vi "Main v1.7.vi"() -> ()   [LabVIEW 2017]
doc: "v0.85:\n- Counts for rejects and total\n\nv0.5:\n\n- Added Reject to Manual Mode\n- Send reject pallet cluster during manual mode\n- Run continuous manual happens only when no error has occured"
uses:
  Controls/Main Tabs v0.1.ctl
  Controls/Auto.ctl
  RT/Controls/Auto Delays.ctl
  RT/Controls/Auto Times.ctl
  support/Controls/General Para.ctl
  support/Message Queue/Message Cluster.ctl
  Controls/UI Data.ctl
  support/Controls/Auto Stats.ctl
  Controls/Logging FGV.ctl
  support/Message Queue/Enqueue Message (Single).vi
  GV/Maintenance GV.vi
  <vilib>/Utility/error.llb/Error Cluster From Error Code.vi
  <vilib>/ErrorRing/Error Ring.xnode
  support/Message Queue/Message Queue.lvlib
  support/User Event - Stop/User Event - Stop.lvlib
panel:
  in  "dup Message Queue":refnum<queue>
  out "path":path
  in  "General Para 2":T1={"Max. Cons."=5.0, "Offset 1"=0.0, "Offset 2"=0.0, "Offset 3"=0.0, "Offset 4"=-0.6, "OutputPause"=500.0, "RejectPause"=500.0} caption="General Para" {"Offset 4" format="%.2f"; "Offset 3" format="%.2f"; "Offset 2" format="%.2f"; "Offset 1" format="%.2f"}
  in  "Auto Para 2":T2={"Agitator Delays"=[250, 600], "TF Delays"=[400, 800, 2, 8000], "Insertion Delays"=[100, 400], "Cutting Delays"=[200, 300, 50], "PF Delays"=[300, 8000], "Measur. Delays"=[200.0, 188.9, 1.0], "Reject Delays"=[500], "BF Delays"=[1000, 1000]}
  out "Shutdown?":bool
  out "Boolean 8":bool
  out "Boolean 7":bool
  out "Boolean 6":bool
  out "Boolean 5":bool
  out "Boolean 4":bool
  out "Boolean 3":bool
  out "Boolean 2":bool
  out "Boolean":bool
  in  "Reject Pallets":T3
  out "Date-Time":string caption="Dip-Tube Assembly Automation (HMI) v1.6"
  out "Main Tab":T4
  in  "All IOs":bool
  in  "Autocycle":T5
  in  "Manual":bool
  in  "Parameters":bool
  in  "Maintenance":bool
  in  "Info":bool
  in  "General Para":T1={"Max. Cons."=5.0, "Offset 1"=0.0, "Offset 2"=0.0, "Offset 3"=0.0, "Offset 4"=0.0, "OutputPause"=0.0, "RejectPause"=0.0} {"Offset 4" format="%.2f"; "Offset 3" format="%.2f"; "Offset 2" format="%.2f"; "Offset 1" format="%.2f"}
  in  "BF Para":cluster{"Delay 1":u32, "Delay 2":u32}={"Delay 1"=1000, "Delay 2"=1000}
  in  "Reject Para":cluster{"Delay":u32}={"Delay"=400}
  in  "Meas. Para":T6={"Delay"=500.0, "Mean Length"=188.9, "Tolerance"=1.0}
  in  "PF Para":cluster{"Delay":u32, "Timeout":u32}={"Delay"=1000, "Timeout"=1000}
  in  "Tube Feeder Para":T7={"Delay"=400, "Delay 2"=250, "Max Attempts"=250, "Timeout"=8000}
  in  "Cutting Para":T8={"Delay"=400, "Delay 2"=250, "Delay 3"=250}
  in  "Agitator Para":cluster{"Delay":u32, "Timeout":u32}={"Delay"=400, "Timeout"=250}
  in  "Insertion Para":cluster{"Delay 1":u32, "Delay 2":u32}={"Delay 1"=1000, "Delay 2"=1000}
  in  "Save Para":bool
  in  "Home Para":bool
  out "OEE":dbl format="%#.1f"
  out "QUA":dbl=100.0 min=0.0 max=100.0 step=0.1
  in  "Ideal Time":dbl=2.0 min=0.0 max=100.0 step=0.1
  in  "AVL":dbl=100.0 min=0.0 max=100.0 step=0.1
  out "Rejects 2":u32 caption="Rejects"
  in  "Reset MCount":bool
  in  "Enable BF?":bool
  in  "Enable Agitate?":bool
  in  "Enable Reject?":bool
  in  "Toggle Motor":bool
  in  "Continuous?":bool
  in  "Enable Measure?":bool
  in  "Enable Index?":bool
  in  "Enable PF?":bool
  in  "Manual Para":T2={"Agitator Delays"=[400, 250], "TF Delays"=[700, 800, 2], "Insertion Delays"=[100, 500], "Cutting Delays"=[300, 300, 100], "PF Delays"=[250, 30000], "Measur. Delays"=[500.0, 188.9, 1.0], "Reject Delays"=[500], "BF Delays"=[1000, 1000]}
  in  "Enable Cutting?":bool
  in  "Enable Insertion?":bool
  in  "Run Manual":bool
  in  "Enable TF?":bool
  in  "Home Manual":bool
  out "Status 2":T10
  out "Measurements":T11 {"Height 1" format="%#.2f"; "Height 2" format="%#.2f"; "Height 3" format="%#.2f"; "Height 4" format="%#.2f"}
  out "Output Count":u32 caption="Output\nCount"
  out "PRF":dbl=100.0 min=0.0 max=100.0 step=0.1
  in  "ResetRejectCount":bool
  in  "ResetGoodCount":bool
  out "RejectPause":u32 caption="Reject Parts"
  out "GoodPause":u32 caption="Good Parts"
  in  "End Cycle":bool
  out "Statuses":string[][](table)
  in  "All IO":bool
  in  "Stats":bool
  in  "Home AC":bool
  out "Status":string
  out "Good":u32 format="%06.0f"
  out "Cycle Time":dbl format="%0.2f"
  out "Rejects":u32 format="%05.0f"
  in  "View Log":bool
  out "Total Count 2":u32 caption="Total Count"
  out "Avg. Time":dbl caption="Avg. Cycle Time (s)" format="%#.3f"
  out "Output Chart":cluster{"Good Parts":u32, "Reject Parts":u32}(graph)
  out "Reject Count":u32
  out "Good Count":u32
  out "Total Time":dbl caption="Effective Cycle Time (s)" format="%#.3f"
  out "Time Chart":T12(graph)
  out "OEE Chart":T13(graph)
  out "Timestamp":string caption="Date & Timestamp"
  out "Latest Measure.":T14 caption="Latest Measurements" {"Length 1 (mm)" format="%#.2f"}
  out "Auto Times":T9
  in  "Back Stats":bool
  out "OEE 2":T13 caption="Latest Measurements" {"AVL" format="%#.1f"; "PRF" format="%#.1f"; "QUA" format="%#.1f"; "OEE" format="%#.1f"}
  out "Measurement Chart":T15(graph)
  in  "Home IOs":bool
  in  "Back IO":bool
  out "IAS 4":dbl format="%#.3f"
  out "IAS 3":dbl format="%#.3f"
  out "IAS 2":dbl format="%#.3f"
  out "IAS 1":dbl format="%#.3f"
  out "DI 1":T16
  out "DI 2":T17
  out "DO 1":T18
  in  "Exit":bool
  in  "Shutdown":bool
  # "HARMONY VISION DIP-TUBE ASSEMBLY AUTOMATION"
  # "Auto-Pause after"
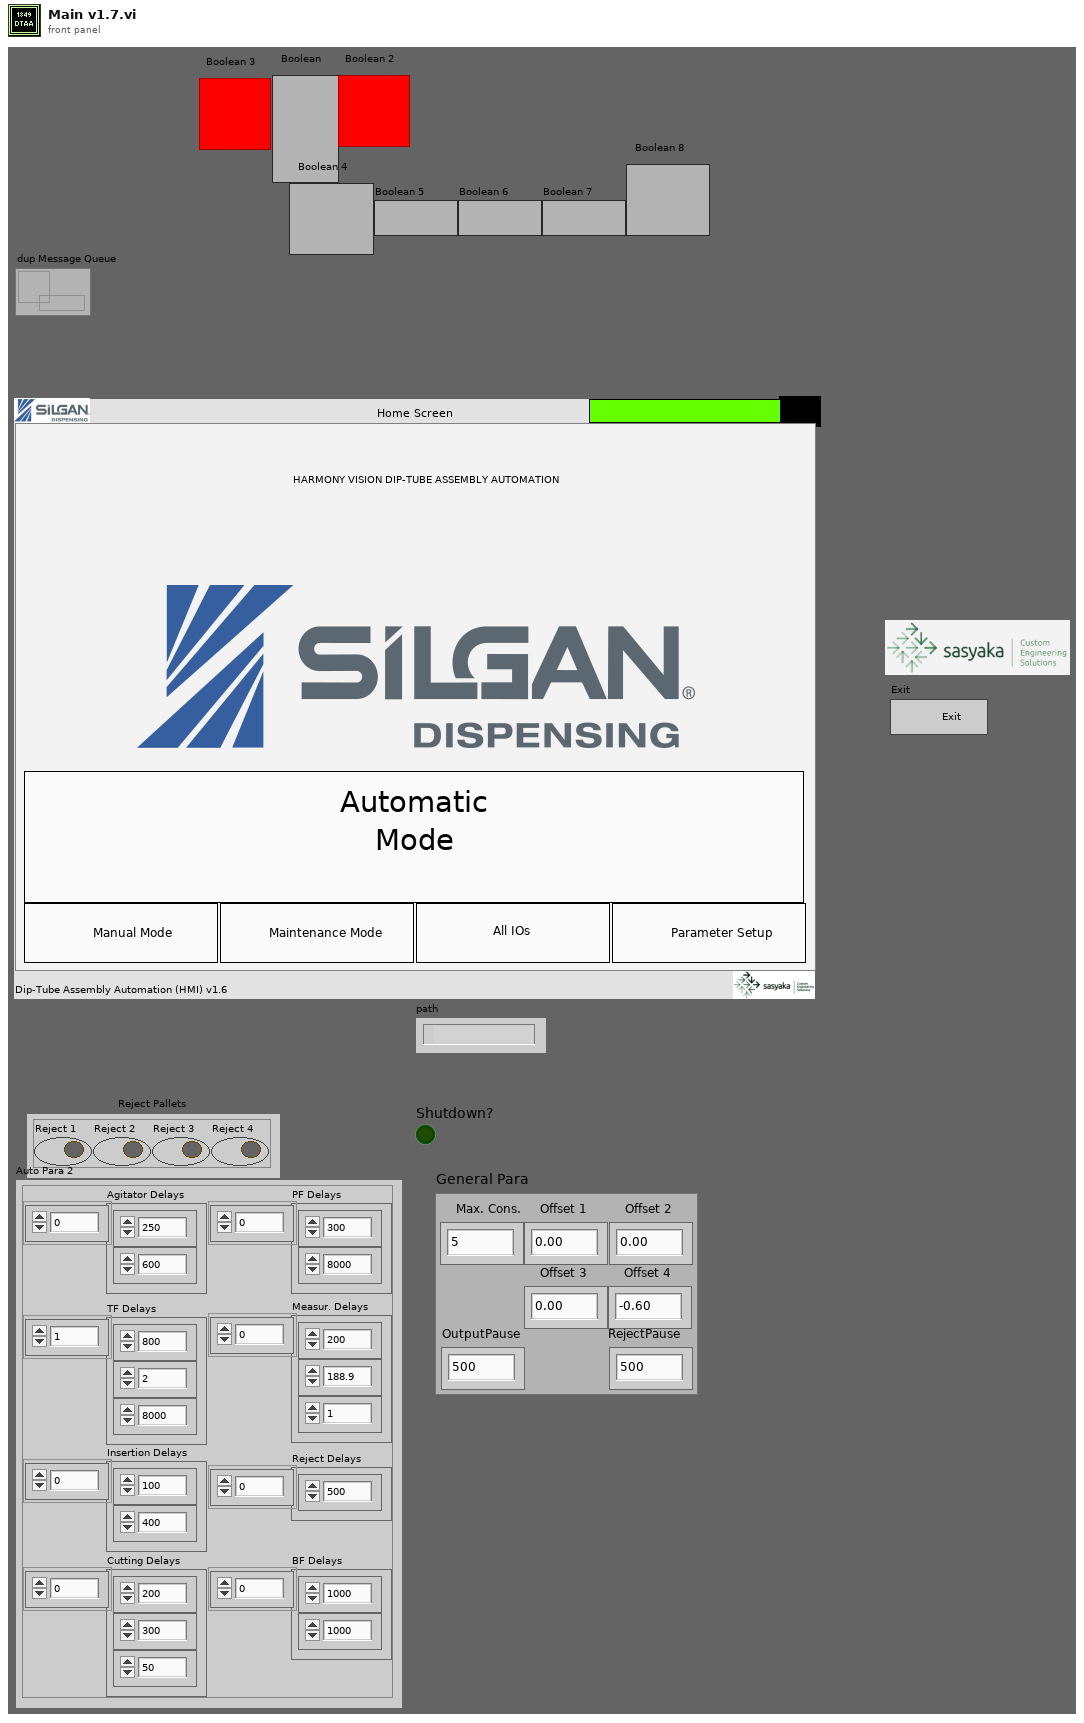
[diagram p1: front panel]
types:
  T1 = typedef "General Para.ctl" = cluster{"Max. Cons.":dbl, "Offset 1":dbl, "Offset 2":dbl, "Offset 3":dbl, "Offset 4":dbl, "OutputPause":dbl, "RejectPause":dbl}
  T2 = typedef "Auto Delays.ctl" = cluster{"Agitator Delays":u32[], "TF Delays":u32[], "Insertion Delays":u32[], "Cutting Delays":u32[], "PF Delays":u32[], "Measur. Delays":dbl[], "Reject Delays":u32[], "BF Delays":u32[]}
  T3 = cluster{"Reject 1":bool, "Reject 2":bool, "Reject 3":bool, "Reject 4":bool}
  T4 = typedef "Main Tabs v0.1.ctl" = enum32{"Home Screen", "Parameter Setup", "Manual Mode", "Autocycle", "Autocycle Statistics", "Autocycle IOs"}
  T5 = typedef "Auto.ctl" = bool
  T6 = cluster{"Delay":dbl, "Mean Length":dbl, "Tolerance":dbl}
  T7 = cluster{"Delay":u32, "Delay 2":u32, "Max Attempts":u32, "Timeout":u32}
  T8 = cluster{"Delay":u32, "Delay 2":u32, "Delay 3":u32}
  T9 = typedef "Auto Times.ctl" = cluster{"Index Time":u32, "TF Time":u32, "Insertion Time":u32, "Cutting Time":u32, "PF Time":u32, "Meas. Time":u32, "Reject Time":u32}
  T10 = cluster{"Auto Times":T9, "error out":errorcluster}
  T11 = cluster{"Height 1":dbl, "Height 2":dbl, "Height 3":dbl, "Height 4":dbl}
  T12 = cluster{"Index":dbl, "TF":dbl, "Insert":dbl, "Cutting":dbl, "PF":dbl, "Measure.":dbl, "Reject":dbl, "Avg. Cycle Time":dbl}
  T13 = cluster{"AVL":dbl, "PRF":dbl, "QUA":dbl, "OEE":dbl}
  T14 = cluster{"Length 1 (mm)":dbl, "Pallet 2 (mm)":dbl, "Pallet 3 (mm)":dbl, "Pallet 4 (mm)":dbl}
  T15 = cluster{"1":dbl, "2":dbl, "3":dbl, "4":dbl, "4":dbl, "4":dbl}
  T16 = cluster{"Machine_ON":bool, "E_stop ":bool, "SW_Pressure":bool, "SW_Start ":bool, "SW_Reset":bool, "SW_Stop":bool, "SW_Door":bool, "RS_Index_Rotary_CW":bool, "RS_Index_Rotary_CCW":bool, "RS_Index_Stopper _Rear":bool, "RS_Index_Output_Separator_Rear":bool, "PES_Index_Pallet_Sensor":bool, "PES_Index_Output_Part Sensor":bool, "ICS_BF_Low_Level_1":bool, "ICS_BF_Low_Level_2":bool, "ICS_BF_Pump_CNVR_Full_1":bool, "ICS_BF_Pump_CNVR_Full_2":bool, "ICS_BF_Pump_CNVR_Full_3":bool, "ICS_BF_Pump_CNVR_Full_4":bool, "PES_PC_Pump Presence_1":bool, "PES_PC_Pump Presence_2":bool, "PES_PC_Pump Presence_3":bool, "PES_PC_Pump Presence_4":bool, "RS_PC_Gating_Front":bool, "PES_Pump_Interference":bool, "PES_TF_Low_Level":bool, "PES_Tube Presence_1":bool, "PES_Tube Presence_2":bool, "PES_Tube Presence_3":bool, "PES_Tube Presence_4":bool, "DI1.30":bool, "DI1.31":bool}
  T17 = cluster{"RS_Agitatator_1_Rear ":bool, "RS_Agitatator_2_Rear ":bool, "RS_TF_Gating CYL_Rear":bool, "RS_Insertion_1_Rear":bool, "RS_Insertion_1_Front":bool, "RS_Insertion _2_Rear":bool, "RS_Insertion _2_Front":bool, "RS_Insertion _3_Rear":bool, "RS_Insertion _3_Front":bool, "RS_Insertion _4_Rear":bool, "RS_Insertion _4_Front":bool, "RS_Insertion_Clamp_Rear":bool, "RS_Cutting_Rear":bool, "RS_Cutting_Clamp _Rear":bool, "RS_Measurement_1_Rear":bool, "RS_Measurement_2_Rear":bool, "RS_Measurement_3_Rear":bool, "RS_Measurement_4_Rear":bool, "DI2.18":bool, "RS_Rejection_1_Rear":bool, "RS_Rejection_2_Rear":bool, "RS_Rejection_3_Rear":bool, "RS_Rejection_4_Rear":bool, "DI2.23":bool, "DI2.24":bool, "DI2.25":bool, "DI2.26":bool, "DI2.27":bool, "DI2.28":bool, "DI2.29":bool, "DI2.30":bool, "DI2.31":bool}
  T18 = cluster{"TL_Red":bool, "TL_Orange":bool, "TL_Green":bool, "TL_Buzzer":bool, "SOL_Index_Rotary_CW":bool, "SOL_Index_Rotary_CCW":bool, "SOL_Index_Stopper_Rear":bool, "SOL_OutputSeparator_Rear":bool, "Bowl  Feeder_ ON 1":bool, "Pump_CNVR_Motor _ON":bool, "SOL_PC_Gating_CYL_Rear":bool, "SOL_Tube_Feed_Agitatator":bool, "SOL_Tube_Feed_Gating_CYL":bool, "SOL_Insertion _CYL":bool, "SOL_Insertion_Clamp_CYL":bool, "SOL_Cutting_CYL":bool, "SOL_Cutting_Clamp_CYL":bool, "SOL_Insertion_Air_Nozzle":bool, "SOL_Measurement_CYL":bool, "DO1.19":bool, "SOL_Rejection CYL_1":bool, "SOL_Rejection CYL_2":bool, "SOL_Rejection CYL_3":bool, "SOL_Rejection CYL_4":bool, "Bowl  Feeder_ ON 2":bool, "SOL_BF_BlowerON":bool, "SOL_BF1_Track1":bool, "SOL_BF1_Track2":bool, "SOL_BF2_Track1":bool, "SOL_BF2_Track2":bool, "DO1.30":bool, "DO1.31":bool}
  T19 = typedef "UI Data.ctl" = cluster{"Main Tab":refnum<vi>}
  T20 = typedef "Message Queue.lvlib/All Message Queues.ctl" = cluster{"UI":refnum<queue>}
  T21 = enum8{"Enabled", "Disabled", "Disabled and Grayed Out"}
  T22 = cluster{"Array":string[][], "Machine Status":string}
  T23 = typedef "Logging FGV.ctl" = enum16{"Start Shift", "Log Index", "Read Shift", "Close Shift"}
  T24 = typedef "Auto Stats.ctl" = cluster{"Time-Stamp":timestamp, "Auto Times":T9, "Measurements":cluster{"1":dbl, "2":dbl, "3":dbl, "4":dbl}, "Outputs":cluster{"Good Parts":u32, "Reject Parts":u32}, "Cycle Time":dbl, "Remarks":string}
  T25 = cluster{"Auto Times":T9, "Results":cluster{"Measurements":cluster{"1":dbl, "2":dbl, "3":dbl, "4":dbl}, "Reject Pallets":cluster{"Reject 1":bool, "Reject 2":bool, "Reject 3":bool, "Reject 4":bool}}, "OutputCount":u32, "error out":errorcluster}
  T26 = enum8{"Information", "Error", "Successful", "Tips"}
  T27 = cluster{"Agitator Delays[0]":u32, "Agitator Delays[1]":u32}
  T28 = cluster{"TF Delays[0]":u32, "TF Delays[1]":u32, "TF Delays[2]":u32, "TF Delays[3]":u32}
  T29 = cluster{"Insertion Delays[0]":u32, "Insertion Delays[1]":u32}
  T30 = cluster{"Cutting Delays[0]":u32, "Cutting Delays[1]":u32, "Cutting Delays[2]":u32}
  T31 = cluster{"Measur. Delays[0]":dbl, "Measur. Delays[1]":dbl, "Measur. Delays[2]":dbl}
  T32 = typedef "All Inputs.ctl" = cluster{"DI 1":cluster{"Machine_ON":bool, "E_stop ":bool, "SW_Pressure":bool, "SW_Start ":bool, "SW_Reset":bool, "SW_Stop":bool, "SW_Door":bool, "RS_Index_Rotary_CW":bool, "RS_Index_Rotary_CCW":bool, "RS_Index_Stopper _Rear":bool, "RS_Cutting_DNClamp _Rear":bool, "PES_Index_Pallet_Sensor":bool, "PES_Index_Output_Part Sensor":bool, "ICS_BF_Low_Level_1":bool, "ICS_BF_Low_Level_2":bool, "ICS_BF_Pump_CNVR_Full_1":bool, "ICS_BF_Pump_CNVR_Full_2":bool, "ICS_BF_Pump_CNVR_Full_3":bool, "ICS_BF_Pump_CNVR_Full_4":bool, "PES_PC_Pump Presence_1":bool, "PES_PC_Pump Presence_2":bool, "PES_PC_Pump Presence_3":bool, "PES_PC_Pump Presence_4":bool, "RS_PC_Gating_Front":bool, "PES_Pump_Interference":bool, "PES_TF_Low_Level":bool, "PES_Tube Presence_1":bool, "PES_Tube Presence_2":bool, "PES_Tube Presence_3":bool, "PES_Tube Presence_4":bool, "DI1.30":bool, "DI1.31":bool}, "DI 2":cluster{"RS_Agitatator_1_Rear ":bool, "RS_Agitatator_2_Rear ":bool, "RS_TF_Gating CYL_Rear":bool, "RS_Insertion_1_Rear":bool, "RS_Insertion_1_Front":bool, "RS_Insertion _2_Rear":bool, "RS_Insertion _2_Front":bool, "RS_Insertion _3_Rear":bool, "RS_Insertion _3_Front":bool, "RS_Insertion _4_Rear":bool, "RS_Insertion _4_Front":bool, "RS_Insertion_Clamp_Rear":bool, "RS_Cutting_Rear":bool, "RS_Cutting_UPClamp _Rear":bool, "RS_Measurement_1_Rear":bool, "RS_Measurement_2_Rear":bool, "RS_Measurement_3_Rear":bool, "RS_Measurement_4_Rear":bool, "RS_Measure_Clamp_Rear":bool, "RS_Rejection_1_Rear":bool, "RS_Rejection_2_Rear":bool, "RS_Rejection_3_Rear":bool, "RS_Rejection_4_Rear":bool, "DI2.23":bool, "DI2.24":bool, "DI2.25":bool, "DI2.26":bool, "DI2.27":bool, "DI2.28":bool, "DI2.29":bool, "DI2.30":bool, "DI2.31":bool}, "IAS 1":dbl, "IAS 2":dbl, "IAS 3":dbl, "IAS 4":dbl, "DO 1":cluster{"TL_Red":bool, "TL_Orange":bool, "TL_Green":bool, "TL_Buzzer":bool, "SOL_Index_Rotary_CW":bool, "SOL_Index_CNVR_Rotary_CCW":bool, "SOL_Index_CNVR_Stopper_Rear":bool, "SOL_Index_CNVR_Output _Separator _Rear":bool, "Bowl  Feeder_ ON 1":bool, "Pump_CNVR_Motor _ON":bool, "SOL_PC_Gating_CYL_Rear":bool, "SOL_Tube_Feed_Agitatator":bool, "SOL_Tube_Feed_Gating_CYL":bool, "SOL_Insertion _CYL":bool, "SOL_Insertion_Clamp_CYL":bool, "SOL_Cutting_CYL":bool, "SOL_Cutting_Clamp_CYL":bool, "SOL_Insertion_Air_Nozzle":bool, "SOL_Measurement_CYL":bool, "DO1.19":bool, "SOL_Rejection CYL_1":bool, "SOL_Rejection CYL_2":bool, "SOL_Rejection CYL_3":bool, "SOL_Rejection CYL_4":bool, "Bowl  Feeder_ ON 2":bool, "SOL_BF_BlowerON":bool, "SOL_BF1_Track1":bool, "SOL_BF1_Track2":bool, "SOL_BF2_Track1":bool, "SOL_BF2_Track2":bool, "DO1.30":bool, "DO1.31":bool}}
  T33 = cluster{"Machine_ON":bool, "E_stop ":bool, "SW_Pressure":bool, "SW_Start ":bool, "SW_Reset":bool, "SW_Stop":bool, "SW_Door":bool, "RS_Index_Rotary_CW":bool, "RS_Index_Rotary_CCW":bool, "RS_Index_Stopper _Rear":bool, "RS_Cutting_DNClamp _Rear":bool, "PES_Index_Pallet_Sensor":bool, "PES_Index_Output_Part Sensor":bool, "ICS_BF_Low_Level_1":bool, "ICS_BF_Low_Level_2":bool, "ICS_BF_Pump_CNVR_Full_1":bool, "ICS_BF_Pump_CNVR_Full_2":bool, "ICS_BF_Pump_CNVR_Full_3":bool, "ICS_BF_Pump_CNVR_Full_4":bool, "PES_PC_Pump Presence_1":bool, "PES_PC_Pump Presence_2":bool, "PES_PC_Pump Presence_3":bool, "PES_PC_Pump Presence_4":bool, "RS_PC_Gating_Front":bool, "PES_Pump_Interference":bool, "PES_TF_Low_Level":bool, "PES_Tube Presence_1":bool, "PES_Tube Presence_2":bool, "PES_Tube Presence_3":bool, "PES_Tube Presence_4":bool, "DI1.30":bool, "DI1.31":bool}
  T34 = cluster{"RS_Agitatator_1_Rear ":bool, "RS_Agitatator_2_Rear ":bool, "RS_TF_Gating CYL_Rear":bool, "RS_Insertion_1_Rear":bool, "RS_Insertion_1_Front":bool, "RS_Insertion _2_Rear":bool, "RS_Insertion _2_Front":bool, "RS_Insertion _3_Rear":bool, "RS_Insertion _3_Front":bool, "RS_Insertion _4_Rear":bool, "RS_Insertion _4_Front":bool, "RS_Insertion_Clamp_Rear":bool, "RS_Cutting_Rear":bool, "RS_Cutting_UPClamp _Rear":bool, "RS_Measurement_1_Rear":bool, "RS_Measurement_2_Rear":bool, "RS_Measurement_3_Rear":bool, "RS_Measurement_4_Rear":bool, "RS_Measure_Clamp_Rear":bool, "RS_Rejection_1_Rear":bool, "RS_Rejection_2_Rear":bool, "RS_Rejection_3_Rear":bool, "RS_Rejection_4_Rear":bool, "DI2.23":bool, "DI2.24":bool, "DI2.25":bool, "DI2.26":bool, "DI2.27":bool, "DI2.28":bool, "DI2.29":bool, "DI2.30":bool, "DI2.31":bool}
  T35 = cluster{"TL_Red":bool, "TL_Orange":bool, "TL_Green":bool, "TL_Buzzer":bool, "SOL_Index_Rotary_CW":bool, "SOL_Index_CNVR_Rotary_CCW":bool, "SOL_Index_CNVR_Stopper_Rear":bool, "SOL_Index_CNVR_Output _Separator _Rear":bool, "Bowl  Feeder_ ON 1":bool, "Pump_CNVR_Motor _ON":bool, "SOL_PC_Gating_CYL_Rear":bool, "SOL_Tube_Feed_Agitatator":bool, "SOL_Tube_Feed_Gating_CYL":bool, "SOL_Insertion _CYL":bool, "SOL_Insertion_Clamp_CYL":bool, "SOL_Cutting_CYL":bool, "SOL_Cutting_Clamp_CYL":bool, "SOL_Insertion_Air_Nozzle":bool, "SOL_Measurement_CYL":bool, "DO1.19":bool, "SOL_Rejection CYL_1":bool, "SOL_Rejection CYL_2":bool, "SOL_Rejection CYL_3":bool, "SOL_Rejection CYL_4":bool, "Bowl  Feeder_ ON 2":bool, "SOL_BF_BlowerON":bool, "SOL_BF1_Track1":bool, "SOL_BF1_Track2":bool, "SOL_BF2_Track1":bool, "SOL_BF2_Track2":bool, "DO1.30":bool, "DO1.31":bool}
  T36 = cluster{"Index":dbl, "TF":dbl, "Insert":dbl, "Cutting":dbl, "PF":dbl, "Measure.":dbl, "Reject":dbl}
  T37 = cluster{"1":dbl, "2":dbl, "3":dbl, "4":dbl, dbl, dbl}
  T38 = cluster{"Manual Para":T2, "Reject Pallets":cluster{"Reject 1":bool, "Reject 2":bool, "Reject 3":bool, "Reject 4":bool}}
  T39 = cluster{"Measurements":cluster{"1":dbl, "2":dbl, "3":dbl, "4":dbl}, "Reject Pallets":cluster{"Reject 1":bool, "Reject 2":bool, "Reject 3":bool, "Reject 4":bool}}
  T40 = cluster{"Reject Pallets":cluster{"Reject 1":bool, "Reject 2":bool, "Reject 3":bool, "Reject 4":bool}, "Measurements":cluster{"1":dbl, "2":dbl, "3":dbl, "4":dbl}}
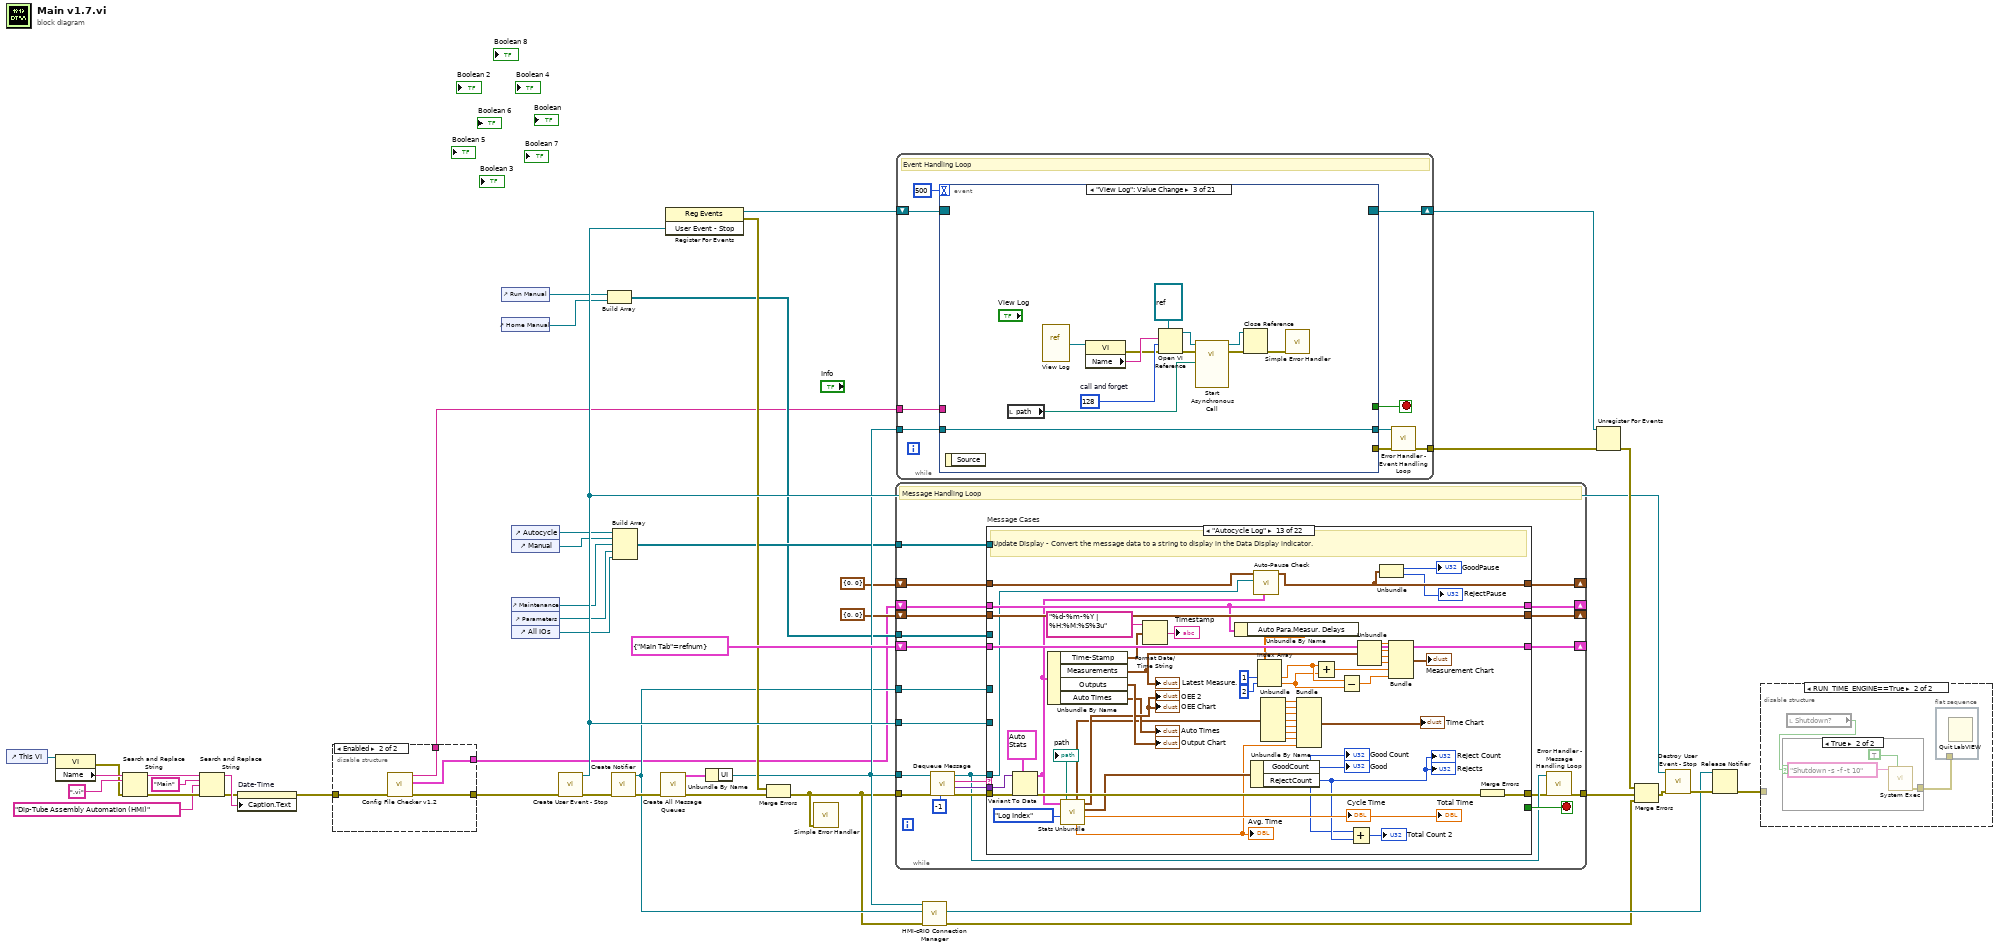
[diagram p0: block diagram]
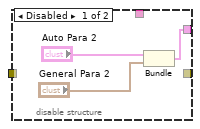
[diagram p2: hidden frame]
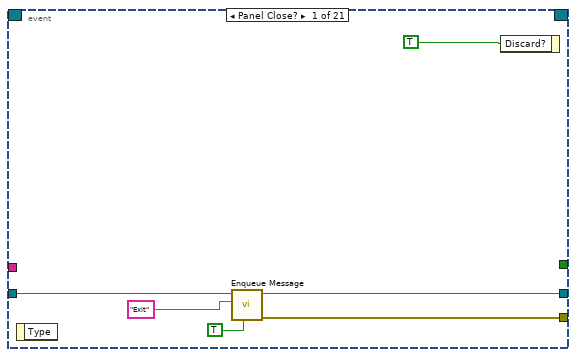
[diagram p3: hidden frame]
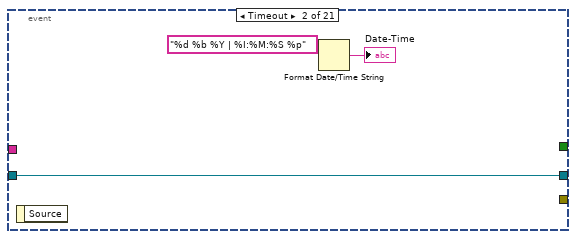
[diagram p4: hidden frame]
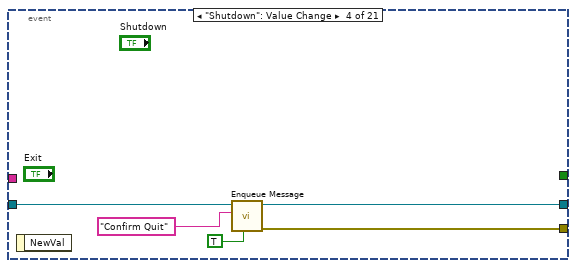
[diagram p5: hidden frame]
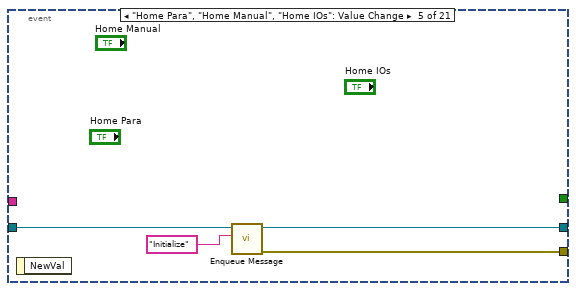
[diagram p6: hidden frame]
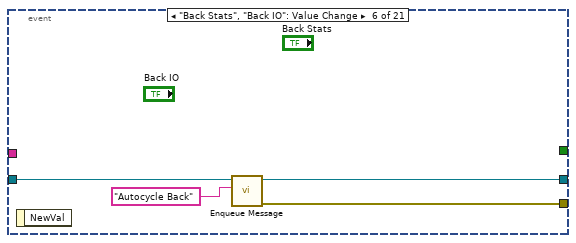
[diagram p7: hidden frame]
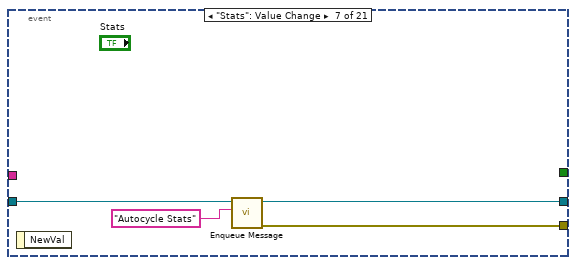
[diagram p8: hidden frame]
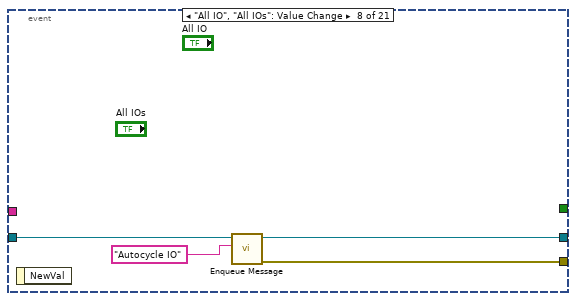
[diagram p9: hidden frame]
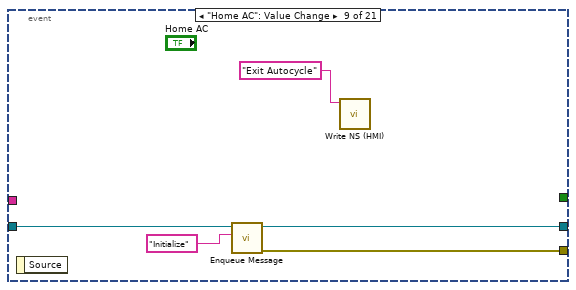
[diagram p10: hidden frame]
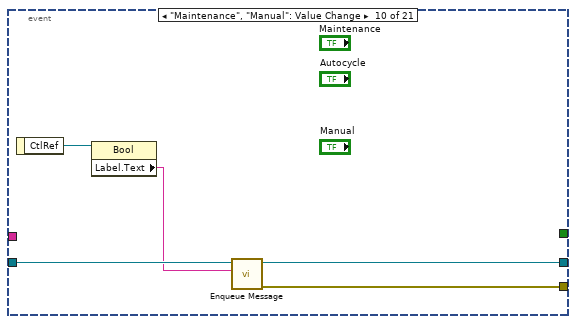
[diagram p11: hidden frame]
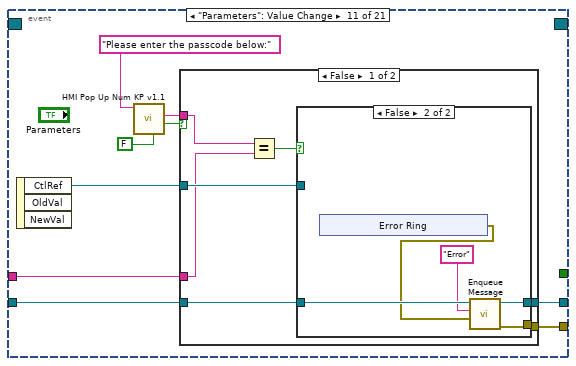
[diagram p12: hidden frame]
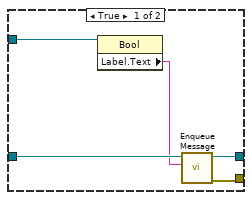
[diagram p13: hidden frame]
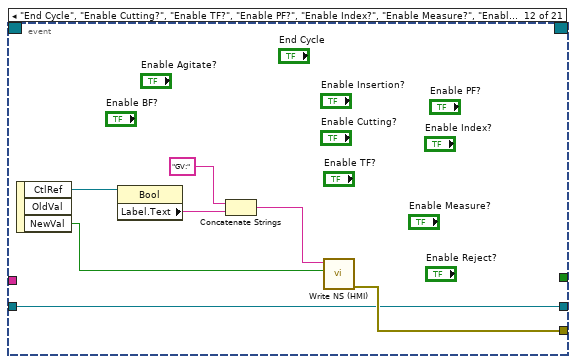
[diagram p15: hidden frame]
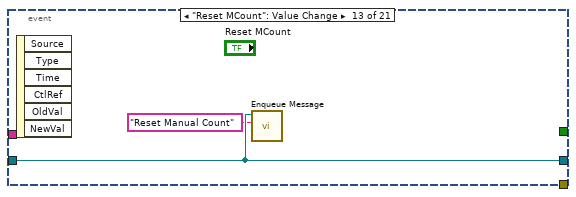
[diagram p16: hidden frame]
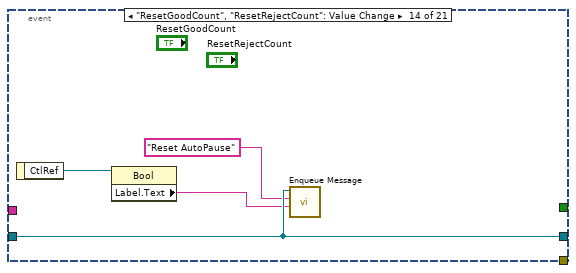
[diagram p17: hidden frame]
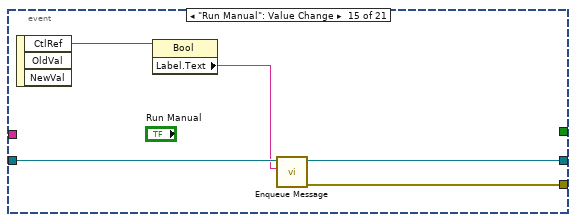
[diagram p18: hidden frame]
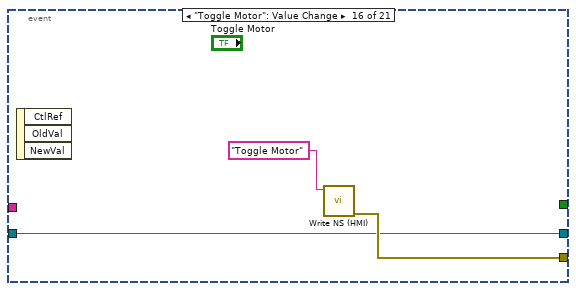
[diagram p19: hidden frame]
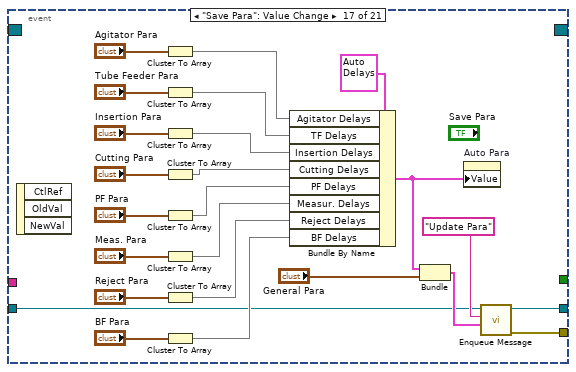
[diagram p20: hidden frame]
diagram:
  n1 = control-ref of="This VI"() -> (w16:refnum<vi>)
  n2 = property class="VI"(reference=w16) -> (error out=w15:errorcluster, "Name"=w22:string)  [unwired: 1 in, 1 out]
  n3 = Search and Replace String(input string=w22, search string=".vi", error in=w15) -> (result string=w20:string, error out=w19:errorcluster)  [unwired: 5 in, 2 out]
  n4 = Search and Replace String(input string=w20, search string="Main", replace string="Dip-Tube Assembly Automation (HMI)" ("replace string (\"\")"), error in=w19) -> (result string=w14:string, error out=w13:errorcluster)  [unwired: 4 in, 2 out]
  n5 = property on="Date-Time" class="Str"(error in=w13, "Caption.Text"=w14) -> (error out=w6:errorcluster)  [unwired: 1 in, 1 out]
  n6 = disable-structure shown="Enabled" {
    disable-tunnel: [w46 w52] -> w4
    disable-tunnel: w6 -> [_ w51]
    disable-tunnel: [_ w50] -> w5
    disable-tunnel: [_ w49] -> w3
    frame Disabled {
      n7 = Bundle("Auto Para 2"="Auto Para 2", "General Para 2"="General Para 2") -> (w46:cluster{"Auto Para 2":T2, "General Para 2":T1})  [unwired: 1 in]
    }
    frame Enabled {
      n8 = call "Config File Checker v1.2.vi"("Error In"=w51) -> ("error out"=w50:errorcluster, "All Para"=w52:cluster{"Auto Para":T2, "General Para 2":T1}, "password"=w49:string)  [unwired: 7 in, 1 out]
    }
  }
  n9 = control-ref of="Run Manual"() -> (w12:refnum<vi>)
  n10 = control-ref of="Home Manual"() -> (w11:refnum<vi>)
  n11 = control-ref of="Autocycle"() -> (w27:refnum<vi>)
  n12 = control-ref of="Manual"() -> (w26:refnum<vi>)
  n13 = control-ref of="Maintenance"() -> (w25:refnum<vi>)
  n14 = control-ref of="Parameters"() -> (w24:refnum<vi>)
  n15 = control-ref of="All IOs"() -> (w7:refnum<vi>)
  n16 = call "Create User Event - Stop.vi"("error in (no error)"=w5) -> ("error out"=w33:errorcluster, "User Event - Stop"=w36:refnum<user-event>)  [unwired: 9 in]
  n17 = Build Array(w12, w11) -> (w10:refnum<vi>[])
  n18 = call "Create Notifier.vi"("error in (no error)"=w33) -> ("error out"=w32:errorcluster, "notifier out"=w8:refnum<notifier>)  [unwired: 9 in]
  n19 = Build Array(w27, w26, w25, w24, w7) -> (w23:refnum<vi>[])
  n20 = call "Create All Message Queues.vi"("error in (no error)"=w32) -> ("error out"=w45:errorcluster, "Message Queues out"=w44:T20)  [unwired: 9 in]
  n21 = register-events(w36) -> (reference out=w37:refnum<event-registration>, error out=w35:errorcluster)  [unwired: 2 in]
  n22 = Unbundle By Name(w44) -> ("UI"=w34:refnum<queue>)
  n23 = Merge Errors(w35, w45) -> (w2:errorcluster)
  n24 = call <vilib>:"Simple Error Handler.vi"("error in (no error)"=w2) -> ()  [unwired: 4 in, 5 out]
  n25 = while {
    tunnel: w34 -> [w67]
    shift-right: [w74] -> _
    shift-left: T19 {"Main Tab"=refnum} ("Data Cluster") -> [w57]
    tunnel: w36 -> [w72]
    tunnel: w2 -> [w71]
    tunnel: [w65] -> w43
    tunnel: w8 -> [w62]
    tunnel: w23 -> [w61]
    tunnel: w10 -> [w60]
    shift-right: [w58] -> _
    shift-left: cluster{"OutputCount":u32, "RejectCount":u32} {"OutputCount"=0, "RejectCount"=0} -> [w59]
    shift-right: [w55] -> _
    shift-left: w4 -> [w56]
    shift-right: [w53] -> _
    shift-left: cluster{"GoodPause":u32, "RejectPause":u32} {"GoodPause"=0, "RejectPause"=0} ("cluster") -> [w54]
    stop <- w73 stop-if-true
    # "Message Handling Loop"
    n26 = call "Dequeue Message.vi"("timeout"=-1, "error in (no error)"=w71, "Message Queue"=w67) -> ("error out"=w70:errorcluster, "Message Data"=w68:variant, "Message"=w69:string, "dup Message Queue"=w66:refnum<queue>)  [unwired: 5 in]
    n27 = case "Message Cases" shown="\"Autocycle Log\"" w69 {
      selector: w69 -> [_ _ _ _ _ _ _ _ _ _ _ _ _ _ _ _ _ _ _ _ _ w487]
      tunnel: w66 -> [_ _ _ _ _ _ _ _ _ w218 w228 _ w273 _ w354 _ _ _ _ w456 w483 _]
      tunnel: w70 -> [w84 w89 w105 w135 w152 w170 w181 w204 w211 w220 w236 w266 w316 w328 w362 w374 w384 w421 w446 w460 w476 _]
      tunnel: [w84 w88 w94 w135 w147 w170 w180 w204 w211 w219 w235 w267 w317 w330 w353 w374 w383 w416 w441 w458 w479 w488] -> w64
      tunnel: w57 -> [w83 w90 w107 w139 w154 w169 w177 w208 w215 w225 w233 w268 w318 w331 w363 w373 w386 w420 w445 w459 w482 w489]
      tunnel: [w82 w90 w107 w139 w154 w169 w177 w208 w215 w225 w233 w268 w318 w331 w363 w373 w386 w420 w445 w459 w482 w489] -> w74
      tunnel: [_ _ _ _ _ _ _ _ _ _ _ _ _ _ _ _ _ _ _ _ TRUE _] -> w73
      tunnel: w68 -> [_ _ w104 _ w151 _ _ _ _ _ _ w265 w315 _ w361 _ w382 w419 w444 _ w473 _]
      tunnel: w72 -> [_ _ _ _ _ _ _ _ _ _ _ _ _ _ _ _ _ _ _ _ w478 _]
      tunnel: w62 -> [_ _ _ _ _ _ _ _ _ _ _ _ _ _ _ _ _ _ _ _ w472 _]
      tunnel: w61 -> [_ _ w100 _ _ _ _ _ _ _ _ _ _ _ _ _ _ _ _ _ _ _]
      tunnel: w60 -> [_ _ _ _ _ _ _ _ _ _ _ _ _ w325 w359 _ _ _ _ _ _ _]
      tunnel: w59 -> [w79 w87 w96 w136 w153 w158 w182 w205 w212 w222 w237 w263 w313 w321 w352 _ w385 w415 w440 w455 w469 w486]
      tunnel: [w79 w87 w96 w136 w153 w158 w182 w205 w212 w222 w237 w263 w313 w321 w347 cluster{"OutputCount":u32, "RejectCount":u32} {"OutputCount"=0, "RejectCount"=0} w385 w415 w440 w455 w469 w486] -> w58
      tunnel: w56 -> [w76 w86 w93 w116 _ w157 w176 w203 w210 w217 w227 w252 w282 w320 w335 w370 w378 w398 w423 w448 w468 w485]
      tunnel: [w76 w86 w93 w116 w146 w157 w176 w203 w210 w217 w227 w252 w282 w320 w335 w370 w378 w398 w423 w448 w468 w485] -> w55
      tunnel: w54 -> [w75 w85 w91 w115 w140 w155 w173 w202 w209 w216 w226 w251 w274 w319 w334 w369 w379 w397 w422 w447 w467 w484]
      tunnel: [w75 w85 w91 w115 w140 w155 w174 w202 w209 w216 w226 w251 w271 w319 w334 w369 w377 w397 w422 w447 w467 w484] -> w53
      frame "Initialize" {
        # "Initialize - All initialization work should take place in this message, since other loops can potentially enqueue messages that execute immediately after this one."
        n28 = control-ref of="Main Tab"() -> (w81:refnum<vi>)
        n29 = Bundle By Name(cluster=w83, "Main Tab"=w81) -> (w82:T19)
        n30 = property on="Home IOs" class="Bool"("Visible"=TRUE) -> ()  [unwired: 2 in, 2 out]
        n31 = property on="Back IO" class="Bool"("Visible"=FALSE) -> ()  [unwired: 2 in, 2 out]
        "Main Tab" <- Main_Tabs_v0.1."Home Screen" ("Main Tab")
      }
      frame "Maintenance" {
        # "Maintenance"
        n32 = call "Maintenance v0.3.vi"("Error In"=w89) -> ("Error out"=w88:errorcluster)  [unwired: 10 in]
      }
      frame "Connection" {
        n33 = Variant To Data(error in=w105, type=FALSE, Variant=w104) -> (data=w92:bool, error out=w95:errorcluster)
        n34 = Select(t=u32 6618880 ("Text.Text Colors:BG Color"), s=w92, f=u32 16762112 ("Text.Text Colors:BG Color")) -> (s? t:f=w101:u32)
        n35 = property on="Date-Time" class="Str"("Text.BGColor"=w101) -> ()  [unwired: 2 in, 2 out]
        n36 = Select(t=T21."Enabled" ("Disabled"), s=w92, f=T21."Disabled and Grayed Out") -> (s? t:f=w98:T21)
        n37 = for {
          tunnel: w100 -> [w114] mode=indexing
          tunnel: w98 -> [w113]
          n38 = property class="Bool"(reference=w114, "DisabledEnum"=w113) -> ()  [unwired: 1 in, 2 out]
        }
        n39 = case shown="True" w92 {
          tunnel: w95 -> [w108 w111]
          tunnel: [w108 w110] -> w94
          tunnel: w93 -> [_ w109]
          frame False {
          }
          frame True {
            n40 = call "Write NS (HMI).vi"("error in (no error)"=w111, "Message Data"=w109, "Message"="Save Para") -> ("error out"=w110:errorcluster)  [unwired: 8 in]
          }
        }
      }
      frame "Parameters" {
        # "Parameters"
        n41 = Unbundle(w116) -> ("Auto Para"=w118:T2, "General Para 2"=w117:T1)
        n42 = Unbundle By Name(w139) -> ("Main Tab"=w138:refnum<vi>)
        n43 = property on="General Para" class="Clust (strict)"("Value"=w117) -> ()  [unwired: 2 in, 2 out]
        n44 = Unbundle(w118) -> ("Agitator Delays"=w134:u32[], "TF Delays"=w133:u32[], "Insertion Delays"=w132:u32[], "Cutting Delays"=w131:u32[], "PF Delays"=w130:u32[], "Measur. Delays"=w129:dbl[], "Reject Delays"=w128:u32[], "BF Delays"=w127:u32[])
        n45 = property class="TabCtl"(reference=w138, "Value"=Main_Tabs_v0.1."Parameter Setup" ("Main Tab")) -> ()  [unwired: 1 in, 2 out]
        n46 = Array To Cluster(array=w134) -> (cluster=w126:T27)
        n47 = Array To Cluster(array=w133) -> (cluster=w125:T28)
        n48 = Array To Cluster(array=w132) -> (cluster=w124:T29)
        n49 = Array To Cluster(array=w131) -> (cluster=w123:T30)
        n50 = Array To Cluster(array=w130) -> (cluster=w122:cluster{"PF Delays[0]":u32, "PF Delays[1]":u32})
        n51 = Array To Cluster(array=w129) -> (cluster=w121:T31)
        n52 = Array To Cluster(array=w128) -> (cluster=w120:cluster{"Reject Delays[0]":u32})
        n53 = Array To Cluster(array=w127) -> (cluster=w119:cluster{"BF Delays[0]":u32, "BF Delays[1]":u32})
        n54 = property on="Agitator Para" class="Clust (strict)"("Value"=w126) -> ()  [unwired: 2 in, 2 out]
        n55 = property on="Tube Feeder Para" class="Clust (strict)"("Value"=w125) -> ()  [unwired: 2 in, 2 out]
        n56 = property on="Insertion Para" class="Clust (strict)"("Value"=w124) -> ()  [unwired: 2 in, 2 out]
        n57 = property on="Cutting Para" class="Clust (strict)"("Value"=w123) -> ()  [unwired: 2 in, 2 out]
        n58 = property on="PF Para" class="Clust (strict)"("Value"=w122) -> ()  [unwired: 2 in, 2 out]
        n59 = property on="Meas. Para" class="Clust (strict)"("Value"=w121) -> ()  [unwired: 2 in, 2 out]
        n60 = property on="Reject Para" class="Clust (strict)"("Value"=w120) -> ()  [unwired: 2 in, 2 out]
        n61 = property on="BF Para" class="Clust (strict)"("Value"=w119) -> ()  [unwired: 2 in, 2 out]
      }
      frame "Update Para" {
        # "Parameters"
        n62 = Variant To Data(error in=w152, type=cluster{"Auto Para":T2, "General Para":T1} {"Auto Para"={"Agitator Delays"=[], "TF Delays"=[], "Insertion Delays"=[], "Cutting Delays"=[], "PF Delays"=[], "Measur. Delays"=[], "Reject Delays"=[], "BF Delays"=[]}, "General Para"={"Max. Cons."=0.0, "Offset 1"=0.0, "Offset 2"=0.0, "Offset 3"=0.0, "Offset 4"=0.0, "OutputPause"=0.0, "RejectPause"=0.0}} ("cluster"), Variant=w151) -> (data=w146:cluster{"Auto Para":T2, "General Para":T1}, error out=w148:errorcluster)
        n63 = call <vilib>:"Application Directory.vi"() -> ("Application Directory"=w145:path)
        n64 = Build Path(base path=w145, name or relative path="data") -> (appended path=w143:path)
        n65 = Build Path(base path=w143, name or relative path="config.ini") -> (appended path=w142:path)
        n66 = call "Write NS (HMI).vi"("error in (no error)"=w148, "Message Data"=w146, "Message"="Save Para") -> ("error out"=w147:errorcluster)  [unwired: 8 in]
        n67 = call "Write Config v1.1.vi"("All Para"=w146, "file path"=w142) -> ()  [unwired: 8 in, 2 out]
      }
      frame "Manual" {
        # "Parameters"
        n68 = control-ref of="Enable Index?"() -> (w166:refnum<vi>)
        n69 = control-ref of="Enable PF?"() -> (w165:refnum<vi>)
        n70 = control-ref of="Enable Cutting?"() -> (w164:refnum<vi>)
        n71 = control-ref of="Enable Insertion?"() -> (w163:refnum<vi>)
        n72 = control-ref of="Enable TF?"() -> (w162:refnum<vi>)
        n73 = control-ref of="Enable Measure?"() -> (w160:refnum<vi>)
        n74 = Unbundle By Name(w157) -> ("Auto Para"=w156:T2)
        n75 = control-ref of="Enable Reject?"() -> (w159:refnum<vi>)
        n76 = Build Array(w166, w165, w164, w163, w162, w160, w159) -> (w161:refnum<vi>[])
        n77 = property on="Auto Para" class="Clust (strict)"("Value"=w156) -> ()  [unwired: 2 in, 2 out]
        n78 = for {
          tunnel: w161 -> [w172] mode=indexing
          n79 = property class="Bool (strict)"(reference=w172, "Val(Sgnl)"=FALSE ("Value (Signaling)")) -> ()  [unwired: 1 in, 2 out]
        }
        n80 = Unbundle By Name(w169) -> ("Main Tab"=w168:refnum<vi>)
        n81 = property class="TabCtl"(reference=w168, "Value"=Main_Tabs_v0.1."Manual Mode" ("Main Tab")) -> ()  [unwired: 1 in, 2 out]
      }
      frame "Autocycle" {
        # "Parameters"
        n82 = call "Select Model v0.1.vi"() -> ("Cancel out"=w178:bool, "Refresh Indicators?"=w175:bool, "Model out"=w179:string)  [unwired: 9 in]
        n83 = case shown="False" w178 {
          tunnel: w181 -> [w191 w201]
          tunnel: [w198 w201] -> w180
          tunnel: w179 -> [w197 _]
          tunnel: w177 -> [w194 _]
          tunnel: w176 -> [w188 _]
          tunnel: w175 -> [_ _]
          tunnel: [w185 w200] -> w174
          tunnel: w173 -> [_ w200]
          frame False {
            n84 = Unbundle By Name(w194) -> ("Main Tab"=w196:refnum<vi>)
            n85 = Unbundle By Name(w188) -> ("General Para 2.OutputPause"=w187:dbl, "General Para 2.RejectPause"=w186:dbl)
            n86 = call "Write NS (HMI).vi"("error in (no error)"=w191, "Message Data"=w188, "Message"="Save Para") -> ("error out"=w190:errorcluster)  [unwired: 8 in]
            n87 = property class="TabCtl"(reference=w196, "Value"=Main_Tabs_v0.1."Autocycle" ("Main Tab")) -> ()  [unwired: 1 in, 2 out]
            n88 = call "Write NS (HMI).vi"("error in (no error)"=w190, "Message Data"=w197, "Message"="Autocycle") -> ("error out"=w198:errorcluster)  [unwired: 8 in]
            n89 = property on="Home IOs" class="Bool"("Visible"=FALSE) -> ()  [unwired: 2 in, 2 out]
            n90 = property on="Back IO" class="Bool"("Visible"=TRUE) -> ()  [unwired: 2 in, 2 out]
            n91 = To Unsigned Long Integer(number=w187) -> (unsigned 32bit integer=w184:u32)
            n92 = To Unsigned Long Integer(number=w186) -> (unsigned 32bit integer=w183:u32)
            n93 = Bundle(w184, w183) -> (w185:cluster{u32, u32})  [unwired: 1 in]
            n94 = local write "GoodPause"(w184) -> ()
            n95 = local write "RejectPause"(w183) -> ()
          }
          frame True {
          }
        }
      }
      frame "Autocycle Back" {
        # "Parameters"
        n96 = Unbundle By Name(w208) -> ("Main Tab"=w207:refnum<vi>)
        n97 = property class="TabCtl"(reference=w207, "Value"=Main_Tabs_v0.1."Autocycle" ("Main Tab")) -> ()  [unwired: 1 in, 2 out]
      }
      frame "Autocycle Stats" {
        # "Parameters"
        n98 = Unbundle By Name(w215) -> ("Main Tab"=w214:refnum<vi>)
        n99 = property class="TabCtl"(reference=w214, "Value"=Main_Tabs_v0.1."Autocycle Statistics" ("Main Tab")) -> ()  [unwired: 1 in, 2 out]
      }
      frame "Autocycle IO" {
        # "Parameters"
        n100 = Unbundle By Name(w225) -> ("Main Tab"=w224:refnum<vi>)
        n101 = property class="TabCtl"(reference=w224, "Value"=Main_Tabs_v0.1."Autocycle IOs" ("Main Tab")) -> ()  [unwired: 1 in, 2 out]
        n102 = call-poly "Enqueue Message.vi"("error in (no error)"=w220, "Message"="Update IO", "Message Queue"=w218) -> ("error out"=w219:errorcluster)  [unwired: 7 in, 1 out]
      }
      frame "Update IO" {
        n103 = Unbundle By Name(w233) -> ("Main Tab"=w234:refnum<vi>)
        n104 = Wait (ms)(milliseconds to wait=u32 200) -> ()  [unwired: 1 out]
        n105 = property class="TabCtl"(reference=w234) -> ("Value"=w232:variant)  [unwired: 1 in, 2 out]
        n106 = Variant To Data(type=Main_Tabs_v0.1."Autocycle IOs" ("Main Tab"), Variant=w232) -> (data=w229:T4)  [unwired: 1 in, 1 out]
        n107 = global read "Maintenance GV.vi" "All IO"() -> (w238:T32)
        n108 = case shown="\"Autocycle IOs\"" w229 {
          tunnel: w236 -> [w246 w249]
          tunnel: [w246 w248] -> w235
          tunnel: w228 -> [_ w247]
          frame Default {
          }
          frame "Autocycle IOs" {
            n109 = call-poly "Enqueue Message.vi"("error in (no error)"=w249, "Message"="Update IO", "Message Queue"=w247) -> ("error out"=w248:errorcluster)  [unwired: 7 in, 1 out]
          }
        }
        n110 = Unbundle(w238) -> ("DI 1"=→"DI 1":T33, "DI 2"=→"DI 2":T34, "IAS 1"=→"IAS 1":dbl, "IAS 2"=→"IAS 2":dbl, "IAS 3"=→"IAS 3":dbl, "IAS 4"=→"IAS 4":dbl, "DO 1"=→"DO 1":T35)
      }
      frame "Update UI" {
        # "Update Display - Convert the message data to a string to display in the Data Display indicator."
        n111 = Variant To Data(error in=w266, type=T22 {"Array"=[], "Machine Status"=""} ("Status Cluster"), Variant=w265) -> (data=w261:T22, error out=w264:errorcluster)
        n112 = Unbundle(w261) -> ("Array"=→"Statuses":string[][], "Machine Status"=w259:string)
        "Status" <- w259
        n113 = Search and Replace String(input string=w259, search string="Autocycle is Running") -> (number of replacements=w257:i32)  [unwired: 6 in, 3 out]
        n114 = Greater Than 0?(x=w257) -> (x > 0?=w255:bool)
        n115 = Select(t=T21."Disabled and Grayed Out" ("Disabled"), s=w255, f=T21."Enabled" ("Disabled")) -> (s? t:f=w254:T21)
        n116 = property on="Home AC" class="Bool"("DisabledEnum"=w254) -> ()  [unwired: 2 in, 2 out]
        n117 = Merge Errors(w264) -> (w267:errorcluster)
      }
      frame "Autocycle Log" {
        # "Update Display - Convert the message data to a string to display in the Data Display indicator."
        n118 = Variant To Data(error in=w316, type=T24 {"Time-Stamp"=timestamp(0 s since 1904-01-01), "Auto Times"={"Index Time"=0, "TF Time"=0, "Insertion Time"=0, "Cutting Time"=0, "PF Time"=0, "Meas. Time"=0, "Reject Time"=0}, "Measurements"={"1"=0.0, "2"=0.0, "3"=0.0, "4"=0.0}, "Outputs"={"Good Parts"=0, "Reject Parts"=0}, "Cycle Time"=0.0, "Remarks"=""} ("Auto Stats"), Variant=w315) -> (data=w272:T24, error out=w314:errorcluster)
        n119 = Unbundle By Name(w272) -> ("Time-Stamp"=w310:timestamp, "Measurements"=w302:cluster{"1":dbl, "2":dbl, "3":dbl, "4":dbl}, "Outputs"=→"Output Chart":cluster{"Good Parts":u32, "Reject Parts":u32}, "Auto Times"=→"Auto Times":T9)
        "Latest Measure." <- w302
        n120 = call "Stats Unbundle.vi"("State"=Logging_FGV."Log Index", "Auto Stats"=w272) -> ("Cycle Time"=→"Cycle Time" →"Total Time":dbl, "Counters"=w306:cluster{"GoodCount":u32, "RejectCount":u32}, "OEE Cluster"=→"OEE Chart" →"OEE 2":T13, "Avg. Cycle Time"=w284:dbl, "Total Times"=w292:T36, "path"=→"path":path)  [unwired: 3 in, 1 out]
        "Avg. Time" <- w284
        n121 = Format Date/Time String(time format string (%c)="%d-%m-%Y | %H:%M:%S%3u", seconds (now)=w310) -> (date/time string=→"Timestamp":string)  [unwired: 1 in]
        n122 = Unbundle By Name(w282) -> ("Auto Para.Measur. Delays"=w281:dbl[])
        n123 = Unbundle By Name(w306) -> ("GoodCount"=w294:u32, "RejectCount"=w295:u32)
        "Rejects" <- w295
        "Good" <- w294
        "Good Count" <- w294
        "Reject Count" <- w295
        n124 = call "Auto-Pause Check.vi"("Auto Stats"=w272, "Queue"=w273, "Autopause"=w274) -> ("Autopause out"=w271:cluster{"GoodPause":u32, "RejectPause":u32})  [unwired: 8 in]
        n125 = Index Array(array=w281, index #1=1 ("index"), index #2=2 ("index")) -> (element #1=w276:dbl, element #2=w275:dbl)
        n126 = Unbundle(w292) -> ("Index"=w291:dbl, "TF"=w290:dbl, "Insert"=w289:dbl, "Cutting"=w288:dbl, "PF"=w287:dbl, "Measure."=w286:dbl, "Reject"=w285:dbl)
        n127 = Bundle("Index"=w291, "TF"=w290, "Insert"=w289, "Cutting"=w288, "PF"=w287, "Measure."=w286, "Reject"=w285, "Avg. Cycle Time"=w284) -> (→"Time Chart":T12)  [unwired: 1 in]
        n128 = Add(x=w276, y=w275) -> (x+y=w278:dbl)
        n129 = Subtract(x=w276, y=w275) -> (x-y=w277:dbl)
        n130 = Add(x=w294, y=w295) -> (x+y=→"Total Count 2":u32)
        n131 = Unbundle(w302) -> ("1"=w301:dbl, "2"=w300:dbl, "3"=w299:dbl, "4"=w298:dbl)
        n132 = Unbundle(w271) -> ("GoodPause"=→"GoodPause":u32, "RejectPause"=→"RejectPause":u32)
        n133 = Bundle("1"=w301, "2"=w300, "3"=w299, "4"=w298, w278, w277) -> (→"Measurement Chart":T37)  [unwired: 1 in]
        n134 = Merge Errors(w314) -> (w317:errorcluster)
      }
      frame "Run Manual" {
        # "Update Manual mode"
        n135 = Bundle("Manual Para"="Manual Para", "Reject Pallets"="Reject Pallets") -> (w322:T38)  [unwired: 1 in]
        n136 = for {
          tunnel: w325 -> [w333] mode=indexing
          tunnel: T21."Disabled and Grayed Out" ("Disabled") -> [w332]
          n137 = property class="Bool"(reference=w333, "DisabledEnum"=w332) -> ()  [unwired: 1 in, 2 out]
        }
        n138 = call "Write NS (HMI).vi"("error in (no error)"=w328, "Message Data"=w322, "Message"="Manual Run") -> ("error out"=w327:errorcluster)  [unwired: 8 in]
        n139 = Merge Errors(w327) -> (w330:errorcluster)
      }
      frame "Manual Status" {
        n140 = Variant To Data(error in=w362, type=T25 {"Auto Times"={"Index Time"=0, "TF Time"=0, "Insertion Time"=0, "Cutting Time"=0, "PF Time"=0, "Meas. Time"=0, "Reject Time"=0}, "Results"={"Measurements"={"1"=0.0, "2"=0.0, "3"=0.0, "4"=0.0}, "Reject Pallets"={"Reject 1"=FALSE, "Reject 2"=FALSE, "Reject 3"=FALSE, "Reject 4"=FALSE}}, "OutputCount"=0, "error out"={"status"=FALSE, "code"=0, "source"=""}} ("cluster"), Variant=w361) -> (data=w358:T25, error out=w353:errorcluster)
        n141 = Unbundle(w358) -> ("Auto Times"=w357:T9, "Results"=w349:T39, "OutputCount"=w348:u32, "error out"=w351:errorcluster)
        n142 = for {
          tunnel: w359 -> [w368] mode=indexing
          tunnel: T21."Enabled" ("Disabled") -> [w367]
          n143 = property class="Bool"(reference=w368, "DisabledEnum"=w367) -> ()  [unwired: 1 in, 2 out]
        }
        n144 = Unbundle(w349) -> ("Measurements"=w337:cluster{"1":dbl, "2":dbl, "3":dbl, "4":dbl}, "Reject Pallets"=w338:T3)
        "Measurements" <- w337
        n145 = Bundle("Auto Times"=w357, "error out"=w351) -> (→"Status 2":T10)  [unwired: 1 in]
        n146 = Bundle("Reject Pallets"=w338, "Measurements"=w337) -> (w336:T40)  [unwired: 1 in]
        n147 = call "Counts Update (manual).vi"("output cluster"=w336, "Desired Cycle Time (s)"="Ideal Time", "AVL"="AVL", "OutputCount"=w348, "Counts in"=w352) -> ("OEE"=w342:T13, "Counts out"=w347:cluster{"OutputCount":u32, "RejectCount":u32})  [unwired: 5 in]
        n148 = Unbundle(w342) -> ("PRF"=→"PRF":dbl, "QUA"=→"QUA":dbl, "OEE"=→"OEE":dbl)  [unwired: 1 out]
        n149 = Unbundle(w347) -> ("OutputCount"=→"Output Count":u32, "RejectCount"=→"Rejects 2":u32)
        n150 = case shown="True" "Continuous?" {
          tunnel: w354 -> [_ w366]
          tunnel: w351 -> [_ w365]
          frame False {
          }
          frame True {
            # "Run if continuous is TRUE & No Error"
            n151 = call-poly "Enqueue Message.vi"("error in (no error)"=w365, "Message"="Run Manual", "Message Queue"=w366) -> ()  [unwired: 7 in, 2 out]
          }
        }
      }
      frame "Reset Manual Count" {
        w371 = u32 0 ("Rejects")
        n152 = local write "Rejects 2"(w371) -> ()
        n153 = local write "Output Count"(w371) -> ()
      }
      frame "Reset AutoPause" {
        n154 = Variant To Data(error in=w384, type="" ("Message"), Variant=w382) -> (data=w380:string, error out=w383:errorcluster)
        n155 = case shown="\"ResetGoodCount\"" w380 {
          tunnel: w379 -> [w391 w396]
          tunnel: [w390 w395] -> w377
          tunnel: w378 -> [w389 w394]
          frame "ResetGoodCount" {
            n156 = Unbundle By Name(w389) -> ("General Para 2.OutputPause"=w388:dbl)
            n157 = To Unsigned Long Integer(number=w388) -> (unsigned 32bit integer=w387:u32)
            n158 = Bundle By Name(cluster=w391, "GoodPause"=w387) -> (w390:cluster{"GoodPause":u32, "RejectPause":u32})
          }
          frame "ResetRejectCount", Default {
            n159 = Unbundle By Name(w394) -> ("General Para 2.RejectPause"=w393:dbl)
            n160 = To Unsigned Long Integer(number=w393) -> (unsigned 32bit integer=w392:u32)
            n161 = Bundle By Name(cluster=w396, "RejectPause"=w392) -> (w395:cluster{"GoodPause":u32, "RejectPause":u32})
          }
        }
        n162 = Unbundle(w377) -> ("GoodPause"=w376:u32, "RejectPause"=w375:u32)
        n163 = local write "GoodPause"(w376) -> ()
        n164 = local write "RejectPause"(w375) -> ()
      }
      frame "Error" {
        w402 = 128  # call and forget
        # "Run async so that this loop will continue to run"
        # "Error"
        n165 = Variant To Data(error in=w421, type=errorcluster {"status"=FALSE, "code"=0, "source"=""} ("error constant"), Variant=w419) -> (data=w414:errorcluster, error out=w417:errorcluster)
        n166 = Unbundle By Name(w414) -> ("source"=w413:string)
        n167 = vi-ref "NewDialog.vi"() -> (w409:refnum<vi>)
        n168 = property class="VI"(reference=w409) -> (error out=w411:errorcluster, "Name"=w410:string)  [unwired: 1 in, 1 out]
        n169 = Search and Replace String(input string=w413, search string="<err>") -> (result string=w401:string)  [unwired: 6 in, 3 out]
        n170 = Open VI Reference(type specifier VI Refnum (for type only)=refnum<vi> refnum, vi path=w410, options=w402, error in (no error)=w411) -> (vi reference=w404:refnum<vi>, error out=w405:errorcluster)  [unwired: 2 in]
        n171 = call-by-ref "Start Asynchronous Call"(reference=w404, error in=w405, "inIcon"=T26."Error", "inTitle"="ERROR", "inMessage"=w401) -> (reference out=w407:refnum<vi>, error out=w406:errorcluster)  [unwired: 6 in, 3 out]
        n172 = Close Reference(reference=w407, error in (no error)=w406) -> (error out=w408:errorcluster)
        n173 = call <vilib>:"Simple Error Handler.vi"("error in (no error)"=w408) -> ()  [unwired: 4 in, 5 out]
        n174 = Merge Errors(w417) -> (w416:errorcluster)
      }
      frame "Reject Pause" {
        w427 = 128  # call and forget
        # "Run async so that this loop will continue to run"
        # "Error"
        n175 = Variant To Data(error in=w446, type=errorcluster {"status"=FALSE, "code"=0, "source"=""} ("error constant"), Variant=w444) -> (data=w439:errorcluster, error out=w442:errorcluster)
        n176 = Unbundle By Name(w439) -> ("source"=w438:string)
        n177 = vi-ref "NewDialog.vi"() -> (w434:refnum<vi>)
        n178 = property class="VI"(reference=w434) -> (error out=w436:errorcluster, "Name"=w435:string)  [unwired: 1 in, 1 out]
        n179 = Search and Replace String(input string=w438, search string="<err>") -> (result string=w426:string)  [unwired: 6 in, 3 out]
        n180 = Open VI Reference(type specifier VI Refnum (for type only)=refnum<vi> refnum, vi path=w435, options=w427, error in (no error)=w436) -> (vi reference=w429:refnum<vi>, error out=w430:errorcluster)  [unwired: 2 in]
        n181 = call-by-ref "Start Asynchronous Call"(reference=w429, error in=w430, "inIcon"=T26."Error", "inTitle"="ERROR", "inMessage"=w426) -> (reference out=w432:refnum<vi>, error out=w431:errorcluster)  [unwired: 6 in, 3 out]
        n182 = Close Reference(reference=w432, error in (no error)=w431) -> (error out=w433:errorcluster)
        n183 = call <vilib>:"Simple Error Handler.vi"("error in (no error)"=w433) -> ()  [unwired: 4 in, 5 out]
        n184 = Merge Errors(w442) -> (w441:errorcluster)
      }
      frame "Confirm Quit" {
        # "Confirm Quit - Message that can confirm whether or not the user wants to exit the application."
        n185 = call "NewDialog.vi"("inIcon"=T26."Information", "inTitle"="SHUTDOWN?", "inButton2Text"="Shutdown", "inButton1Text"="", "inMessage"="Are you sure you want to shutdown?") -> ("outButton2"=w449:bool)  [unwired: 4 in, 2 out]
        "Shutdown?" <- w449
        n186 = case shown="True" w449 {
          tunnel: w460 -> [w461 w466]
          tunnel: [w461 w465] -> w457
          tunnel: w456 -> [_ w464]
          frame False {
          }
          frame True {
            n187 = call-poly "Enqueue Message.vi"("Priority Message? (F)"=TRUE, "error in (no error)"=w466, "Message"="Exit", "Message Queue"=w464) -> ("error out"=w465:errorcluster)  [unwired: 6 in, 1 out]
          }
        }
        n188 = Merge Errors(w457) -> (w458:errorcluster)
      }
      frame "Exit" {
        # "Stop the VI"
        # "Release the message queue reference"
        # "Exit - Exit the application."
        n189 = Variant To Data(type=errorcluster {"status"=FALSE, "code"=0, "source"=""} ("error constant"), Variant=w473) -> (data=w474:errorcluster)  [unwired: 1 in, 1 out]
        n190 = call <vilib>:"Simple Error Handler.vi"("error in (no error)"=w474) -> ()  [unwired: 4 in, 5 out]
        n191 = Send Notification(notification=TRUE, notifier=w472) -> (error out=w470:errorcluster)  [unwired: 1 in, 1 out]
        n192 = call "Fire User Event - Stop.vi"("User Event - Stop"=w478) -> ("error out"=w477:errorcluster)  [unwired: 10 in]
        n193 = Release Queue(queue=w483, error in (no error)=w476) -> (error out=w480:errorcluster)  [unwired: 1 in, 2 out]
        n194 = Merge Errors(w470, w477, w480) -> (w479:errorcluster)
      }
      frame Default {
        # "'Default' case only runs if there is a message that isn't defined in any of the other cases.  Output a programming error."
        n195 = xnode "Error Ring"("parameter 0"=w487) -> ("error out"=w488:errorcluster)
      }
    }
    n196 = call "Error Handler - Message Handling Loop.vi"("error in (no error)"=w64, "Message Queue"=w66) -> ("dup error in"=w65:errorcluster)  [unwired: 8 in, 1 out]
  }
  n197 = while {
    tunnel: w34 -> [w505]
    shift-right: [w503] -> w40
    shift-left: w37 -> [w504]
    tunnel: [w499] -> w38
    tunnel: w3 -> [w497]
    stop <- w501 stop-if-true
    # "Event Handling Loop"
    n198 = event shown="[2] \"View Log\": Value Change" {
      selector: w504 -> [_ _ _ _ _ _ _ _ _ _ _ _ _ _ _ _ _ _ _ _ _]
      dyn-events: [_ _ _ _ _ _ _ _ _ _ _ _ _ _ _ _ _ _ _ _ _] -> w503
      timeout: 500 -> [_ _ _ _ _ _ _ _ _ _ _ _ _ _ _ _ _ _ _ _ _]
      tunnel: [_ _ _ _ _ _ _ _ _ _ _ _ _ _ _ _ _ _ _ _ TRUE ("Discard?")] -> w501
      tunnel: w505 -> [w510 w514 w526 w531 w535 w539 w543 w547 w552 w557 w566 w590 w594 w598 w603 w605 w608 w639 w648 w657 w659]
      tunnel: [w509 _ _ w530 w534 w538 w542 w546 w551 w556 w565 w591 _ _ w601 w606 w611 _ _ _ _] -> w502
      tunnel: [w508 w514 w526 w529 w533 w537 w541 w545 w550 w555 w564 w590 w594 w598 w602 w605 w607 w639 w648 w657 w659] -> w500
      tunnel: w497 -> [_ _ _ _ _ _ _ _ _ _ w558 _ _ _ _ _ _ _ _ _ _]
      event Panel Close? {
        n199 = event-data() -> ()  [unwired: 1 in, 1 out]
        n200 = call-poly "Enqueue Message.vi"("Priority Message? (F)"=TRUE, "Message"="Exit", "Message Queue"=w510) -> ("error out"=w509:errorcluster, "dup Message Queue"=w508:refnum<queue>)  [unwired: 7 in]
        n201 = event-data("Discard?"=TRUE) -> ()  [unwired: 1 in, 1 out]
      }
      event Timeout {
        n202 = event-data() -> ()  [unwired: 1 in, 1 out]
        n203 = Format Date/Time String(time format string (%c)="%d %b %Y | %I:%M:%S %p") -> (date/time string=→"Date-Time":string)  [unwired: 2 in]
      }
      event "View Log": Value Change {
        w525 = 128  # call and forget
        n204 = event-data() -> ()  [unwired: 1 in, 1 out]
        n205 = local read "path"() -> (w515:path)
        n206 = vi-ref "View Log.vi"() -> (w518:refnum<vi>)
        n207 = property class="VI"(reference=w518) -> (error out=w516:errorcluster, "Name"=w517:string)  [unwired: 1 in, 1 out]
        n208 = Open VI Reference(type specifier VI Refnum (for type only)=refnum<vi> refnum, vi path=w517, options=w525, error in (no error)=w516) -> (vi reference=w523:refnum<vi>, error out=w522:errorcluster)  [unwired: 2 in]
        n209 = call-by-ref "Start Asynchronous Call"(reference=w523, error in=w522, "file path"=w515) -> (reference out=w520:refnum<vi>, error out=w521:errorcluster)  [unwired: 10 in, 1 out]
        n210 = Close Reference(reference=w520, error in (no error)=w521) -> (error out=w519:errorcluster)
        n211 = call <vilib>:"Simple Error Handler.vi"("error in (no error)"=w519) -> ()  [unwired: 4 in, 5 out]
      }
      event "Shutdown": Value Change {
        n212 = event-data() -> ()  [unwired: 1 in, 1 out]
        n213 = call-poly "Enqueue Message.vi"("Priority Message? (F)"=TRUE, "Message"="Confirm Quit", "Message Queue"=w531) -> ("error out"=w530:errorcluster, "dup Message Queue"=w529:refnum<queue>)  [unwired: 7 in]
      }
      event "Home Para", "Home Manual", "Home IOs": Value Change {
        n214 = event-data() -> ()  [unwired: 1 in, 1 out]
        n215 = call-poly "Enqueue Message.vi"("Message"="Initialize", "Message Queue"=w535) -> ("error out"=w534:errorcluster, "dup Message Queue"=w533:refnum<queue>)  [unwired: 8 in]
      }
      event "Back Stats", "Back IO": Value Change {
        n216 = event-data() -> ()  [unwired: 1 in, 1 out]
        n217 = call-poly "Enqueue Message.vi"("Message"="Autocycle Back", "Message Queue"=w539) -> ("error out"=w538:errorcluster, "dup Message Queue"=w537:refnum<queue>)  [unwired: 8 in]
      }
      event "Stats": Value Change {
        n218 = event-data() -> ()  [unwired: 1 in, 1 out]
        n219 = call-poly "Enqueue Message.vi"("Message"="Autocycle Stats", "Message Queue"=w543) -> ("error out"=w542:errorcluster, "dup Message Queue"=w541:refnum<queue>)  [unwired: 8 in]
      }
      event "All IO", "All IOs": Value Change {
        n220 = event-data() -> ()  [unwired: 1 in, 1 out]
        n221 = call-poly "Enqueue Message.vi"("Message"="Autocycle IO", "Message Queue"=w547) -> ("error out"=w546:errorcluster, "dup Message Queue"=w545:refnum<queue>)  [unwired: 8 in]
      }
      event "Home AC": Value Change {
        n222 = event-data() -> ()  [unwired: 1 in, 1 out]
        n223 = call-poly "Enqueue Message.vi"("Message"="Initialize", "Message Queue"=w552) -> ("error out"=w551:errorcluster, "dup Message Queue"=w550:refnum<queue>)  [unwired: 8 in]
        n224 = call "Write NS (HMI).vi"("Message"="Exit Autocycle") -> ()  [unwired: 10 in, 1 out]
      }
      event "Maintenance", "Manual": Value Change {
        n225 = event-data() -> ("CtlRef"=w554:refnum<vi>)  [unwired: 1 in]
        n226 = property class="Bool"(reference=w554) -> ("Label.Text"=w553:string)  [unwired: 1 in, 2 out]
        n227 = call-poly "Enqueue Message.vi"("Message"=w553, "Message Queue"=w557) -> ("error out"=w556:errorcluster, "dup Message Queue"=w555:refnum<queue>)  [unwired: 8 in]
      }
      event "Parameters": Value Change {
        n228 = event-data() -> ("CtlRef"=w563:refnum<vi>)  [unwired: 1 in, 2 out]
        n229 = call "HMI Pop Up Num KP v1.1.vi"("Password Display (F)"=FALSE, "Message In"="Please enter the passcode below:") -> ("Canceled"=w560:bool, "String Out"=w559:string)  [unwired: 8 in]
        n230 = case shown="False" w560 {
          tunnel: w566 -> [w573 w585]
          tunnel: [w572 _] -> w565
          tunnel: [w571 w585] -> w564
          tunnel: w563 -> [w570 _]
          tunnel: w559 -> [w569 _]
          tunnel: w558 -> [w568 _]
          frame False {
            n231 = Equal?(x=w569, y=w568) -> (x = y?=w567:bool)
            n232 = case shown="False" w567 {
              tunnel: w573 -> [w578 w583]
              tunnel: [w577 w582] -> w572
              tunnel: [w576 w581] -> w571
              tunnel: w570 -> [w575 _]
              frame True {
                n233 = property class="Bool"(reference=w575) -> ("Label.Text"=w574:string)  [unwired: 1 in, 2 out]
                n234 = call-poly "Enqueue Message.vi"("Message"=w574, "Message Queue"=w578) -> ("error out"=w577:errorcluster, "dup Message Queue"=w576:refnum<queue>)  [unwired: 8 in]
              }
              frame False {
                n235 = xnode "Error Ring"() -> ("error out"=w579:errorcluster)
                n236 = call-poly "Enqueue Message.vi"("Message Data"=w579, "Message"="Error" ("Message In"), "Message Queue"=w583) -> ("error out"=w582:errorcluster, "dup Message Queue"=w581:refnum<queue>)  [unwired: 7 in]
              }
            }
          }
          frame True {
          }
        }
      }
      event "End Cycle", "Enable Cutting?", "Enable TF?", "Enable PF?", "Enable Index?", "Enable Measure?", "Enable Reject?", "Enable Agitate?", "Enable BF?", "Enable Insertion?": Value Change {
        n237 = event-data() -> ("CtlRef"=w592:refnum<vi>, "NewVal"=w586:bool)  [unwired: 1 in, 1 out]
        n238 = property class="Bool"(reference=w592) -> ("Label.Text"=w589:string)  [unwired: 1 in, 2 out]
        n239 = Concatenate Strings("GV:" ("string"), w589) -> (w587:string)
        n240 = call "Write NS (HMI).vi"("Message Data"=w586, "Message"=w587) -> ("error out"=w591:errorcluster)  [unwired: 9 in]
      }
      event "Reset MCount": Value Change {
        n241 = event-data() -> ()  [unwired: 1 in, 6 out]
        n242 = call-poly "Enqueue Message.vi"("Message"="Reset Manual Count", "Message Queue"=w594) -> ()  [unwired: 8 in, 2 out]
      }
      event "ResetGoodCount", "ResetRejectCount": Value Change {
        n243 = event-data() -> ("CtlRef"=w596:refnum<vi>)  [unwired: 1 in]
        n244 = property class="Bool"(reference=w596) -> ("Label.Text"=w595:string)  [unwired: 1 in, 2 out]
        n245 = call-poly "Enqueue Message.vi"("Message Data"=w595, "Message"="Reset AutoPause", "Message Queue"=w598) -> ()  [unwired: 7 in, 2 out]
      }
      event "Run Manual": Value Change {
        n246 = event-data() -> ("CtlRef"=w600:refnum<vi>)  [unwired: 1 in, 2 out]
        n247 = property class="Bool"(reference=w600) -> ("Label.Text"=w599:string)  [unwired: 1 in, 2 out]
        n248 = call-poly "Enqueue Message.vi"("Message"=w599, "Message Queue"=w603) -> ("error out"=w601:errorcluster, "dup Message Queue"=w602:refnum<queue>)  [unwired: 8 in]
      }
      event "Toggle Motor": Value Change {
        n249 = event-data() -> ()  [unwired: 1 in, 3 out]
        n250 = call "Write NS (HMI).vi"("Message"="Toggle Motor") -> ("error out"=w606:errorcluster)  [unwired: 10 in]
      }
      event "Save Para": Value Change {
        n251 = event-data() -> ()  [unwired: 1 in, 3 out]
        n252 = Cluster To Array(cluster="Agitator Para") -> (array=w628:u32[])
        n253 = Cluster To Array(cluster="Tube Feeder Para") -> (array=w626:u32[])
        n254 = Cluster To Array(cluster="Insertion Para") -> (array=w624:u32[])
        n255 = Cluster To Array(cluster="Cutting Para") -> (array=w622:u32[])
        n256 = Cluster To Array(cluster="PF Para") -> (array=w620:u32[])
        n257 = Cluster To Array(cluster="Meas. Para") -> (array=w618:dbl[])
        n258 = Cluster To Array(cluster="Reject Para") -> (array=w616:u32[])
        n259 = Cluster To Array(cluster="BF Para") -> (array=w614:u32[])
        n260 = Bundle By Name(cluster=T2 {"Agitator Delays"=[1000], "TF Delays"=[1000], "Insertion Delays"=[1000], "Cutting Delays"=[1000], "PF Delays"=[1000], "Measur. Delays"=[1000.0], "Reject Delays"=[1000], "BF Delays"=[1000]} ("Auto Para"), "Agitator Delays"=w628, "TF Delays"=w626, "Insertion Delays"=w624, "Cutting Delays"=w622, "PF Delays"=w620, "Measur. Delays"=w618, "Reject Delays"=w616, "BF Delays"=w614) -> (w613:T2)
        n261 = Bundle("Auto Para"=w613, "General Para"="General Para") -> (w610:cluster{"Auto Para":T2, "General Para":T1})  [unwired: 1 in]
        n262 = property on="Auto Para" class="Clust (strict)"("Value"=w613) -> ()  [unwired: 2 in, 2 out]
        n263 = call-poly "Enqueue Message.vi"("Message Data"=w610, "Message"="Update Para", "Message Queue"=w608) -> ("error out"=w611:errorcluster, "dup Message Queue"=w607:refnum<queue>)  [unwired: 7 in]
      }
      event "Insertion Para.Delay 1", "Insertion Para.Delay 2", "Agitator Para.Delay", "Agitator Para.Timeout", "Cutting Para.Delay", "Cutting Para.Delay 2", "Cutting Para.Delay 3", "Tube Feeder Para.Delay", "Tube Feeder Para.Delay 2", "Tube Feeder Para.Max Attempts", "PF Para.Delay", "PF Para.Timeout", "Reject Para.Delay", "BF Para.Delay 1", "BF Para.Delay 2", "Tube Feeder Para.Timeout": Mouse Up {
        n264 = event-data() -> ("CtlRef"=w631:refnum<vi>)  [unwired: 1 in, 4 out]
        n265 = property class="DigNum (strict)"(reference=w631) -> (reference out=w634:refnum<vi>, "Value"=w635:u32)  [unwired: 1 in, 1 out]
        n266 = Number To Fractional String(number=w635, precision (6)=0.0 ("width (-)")) -> (F-format string=w633:string)  [unwired: 2 in]
        n267 = call "HMI Pop Up Num KP v1.1.vi"("String In"=w633) -> ("String Out"=w632:string)  [unwired: 9 in, 1 out]
        n268 = Fract/Exp String To Number(string=w632, default (0 dbl)=0.0 ("default (0 I32)")) -> (number=w637:dbl)  [unwired: 2 in, 1 out]
        n269 = property class="DigNum (strict)"(reference=w634, "Value"=w637) -> ()  [unwired: 1 in, 2 out]
      }
      event "Meas. Para.Delay": Mouse Up {
        n270 = event-data() -> ("CtlRef"=w640:refnum<vi>)  [unwired: 1 in, 4 out]
        n271 = property class="DigNum (strict)"(reference=w640) -> (reference out=w643:refnum<vi>, "Value"=w644:dbl)  [unwired: 1 in, 1 out]
        n272 = Number To Fractional String(number=w644, precision (6)=0.0 ("width (-)")) -> (F-format string=w642:string)  [unwired: 2 in]
        n273 = call "HMI Pop Up Num KP v1.1.vi"("String In"=w642) -> ("String Out"=w641:string)  [unwired: 9 in, 1 out]
        n274 = Fract/Exp String To Number(string=w641, default (0 dbl)=0.0 ("default (0 I32)")) -> (number=w646:dbl)  [unwired: 2 in, 1 out]
        n275 = property class="DigNum (strict)"(reference=w643, "Value"=w646) -> ()  [unwired: 1 in, 2 out]
      }
      event "Meas. Para.Mean Length", "Meas. Para.Tolerance": Mouse Up {
        n276 = event-data() -> ("CtlRef"=w649:refnum<vi>)  [unwired: 1 in, 4 out]
        n277 = property class="DigNum (strict)"(reference=w649) -> (reference out=w652:refnum<vi>, "Value"=w653:dbl)  [unwired: 1 in, 1 out]
        n278 = Number To Fractional String(number=w653, precision (6)=2.0 ("width (-)")) -> (F-format string=w651:string)  [unwired: 2 in]
        n279 = call "HMI Pop Up Num KP v1.1.vi"("String In"=w651) -> ("String Out"=w650:string)  [unwired: 9 in, 1 out]
        n280 = Fract/Exp String To Number(string=w650, default (0 dbl)=0.0 ("default (0 I32)")) -> (number=w655:dbl)  [unwired: 2 in, 1 out]
        n281 = property class="DigNum (strict)"(reference=w652, "Value"=w655) -> ()  [unwired: 1 in, 2 out]
      }
      event User Event {
        # "The Message Handling Loop processed an \"Exit\" message, which fired this event to stop the Event Handling Loop."
        n282 = event-data() -> ()  [unwired: 1 in, 1 out]
      }
    }
    n283 = call "Error Handler - Event Handling Loop.vi"("error in (no error)"=w502, "Message Queue"=w500) -> ("dup error in"=w499:errorcluster)  [unwired: 8 in, 1 out]
  }
  n284 = call "HMI-cRIO Connection Manager.vi"("error in"=w2, "notifier in"=w8, "Queue in"=w34) -> ("error out"=w28:errorcluster, "Notifier out"=w29:refnum<notifier>)  [unwired: 7 in]
  n285 = Unregister For Events(event registration refnum=w40, error in=w38) -> (error out=w41:errorcluster)
  n286 = Merge Errors(w41, w43, w28) -> (w42:errorcluster)
  n287 = call "Destroy User Event - Stop.vi"("error in (no error)"=w42, "User Event - Stop"=w36) -> ("error out"=w31:errorcluster)  [unwired: 9 in]
  n288 = Release Notifier(notifier=w29, error in (no error)=w31) -> (error out=w30:errorcluster)  [unwired: 1 in, 2 out]
  n289 = disable-structure shown="RUN_TIME_ENGINE==True" {
    disable-tunnel: w30 -> [_ _]
    frame condition #0 (active) {
    }
    frame condition #1 {
      n290 = local read "Shutdown?"() -> (w660:bool)
      n291 = case shown="True" w660 {
        tunnel: [_ w662] -> w661
        frame False {
        }
        frame True {
          n292 = call <vilib>:"System Exec.vi"("wait until completion? (T)"=TRUE, "command line"="Shutdown -s -f -t 10") -> ("error out"=w662:errorcluster)  [unwired: 6 in, 3 out]
        }
      }
      n293 = flat-sequence {
        tunnel: w661 -> [_]
        frame #0 {
          n294 = Quit LabVIEW() -> ()  [unwired: 1 in]
        }
      }
    }
  }
